vi "station_keeping_details.vi"(8 "error in (no error)":errorcluster, 11 "Mission in":refnum<class "Mission.lvclass">) -> (0 "error out":errorcluster, 1 "Buoy SE":cluster{"X":dbl, "Y":dbl}, 2 "Buoy NE":cluster{"X":dbl, "Y":dbl}, 3 "Mission out":refnum<class "Mission.lvclass">, 4 "Buoy SW":cluster{"X":dbl, "Y":dbl}, 5 "Buoy NW":cluster{"X":dbl, "Y":dbl})   [LabVIEW 2011, in "Mission.lvclass"]
uses:
  Mission.lvclass
  Mission.lvclass/Mission.ctl
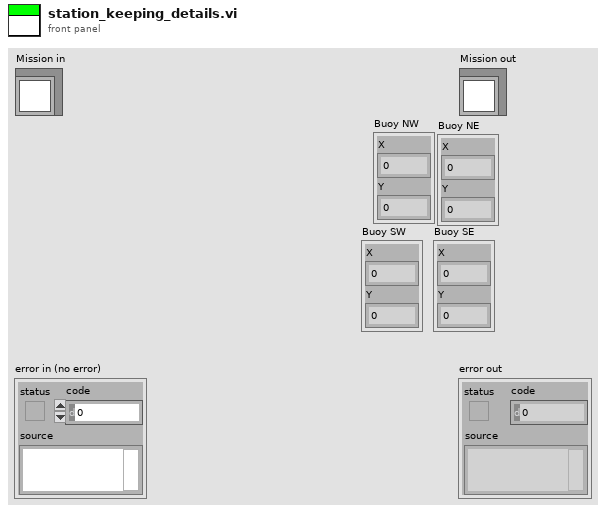
[diagram p1: front panel]
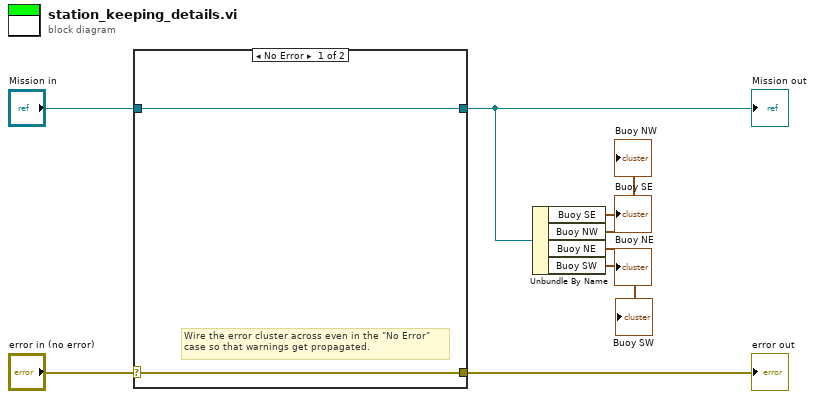
[diagram p0: block diagram]
diagram:
  n1 = case shown="No Error" "error in (no error)" {
    selector: "error in (no error)" -> [w9 w12]
    tunnel: [w9 w12] -> w7
    tunnel: [w10 w11] -> w5
    tunnel: "Mission in" -> [w10 w11]
    frame No Error {
      # "Wire the error cluster across even in the \"No Error\"\ncase so that warnings get propagated."
    }
    frame Error {
    }
  }
  "error out" <- w7
  "Mission out" <- w5
  n2 = Unbundle By Name(w5) -> ("Buoy SE"=→"Buoy SE":cluster{"X":dbl, "Y":dbl}, "Buoy NW"=→"Buoy NW":cluster{"X":dbl, "Y":dbl}, "Buoy NE"=→"Buoy NE":cluster{"X":dbl, "Y":dbl}, "Buoy SW"=→"Buoy SW":cluster{"X":dbl, "Y":dbl})
